vi "Digital In Test_TS_v2.vi"(8 "error in (no error)":errorcluster, 11 "ControlBoard VISA":refnum<visa-resource-name>="ControlBoard") -> (0 "error out":errorcluster, 2 "Message OUT":string, 3 "Result (bool)":bool)   [LabVIEW 2022 SP3]
uses:
  <vilib>/DAQmx/write.llb/DAQmx Write (Digital 1D Bool NChan 1Samp 1Line).vi
  <vilib>/DAQmx/miscellaneous.llb/DAQmx Fill In Error Info.vi
panel:
  in  "Message IN":string
  out "cDAQ DO Cmd":bool[](array[boolean])
  out "DI Reading":bool[](array[boolean])
  out "ControlBoard VISA Out":refnum<visa-resource-name>
  out "Result (color)":u32(colorbox)
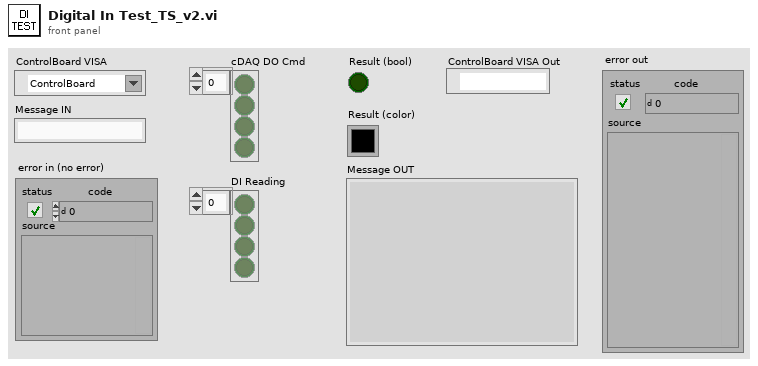
[diagram p1: front panel]
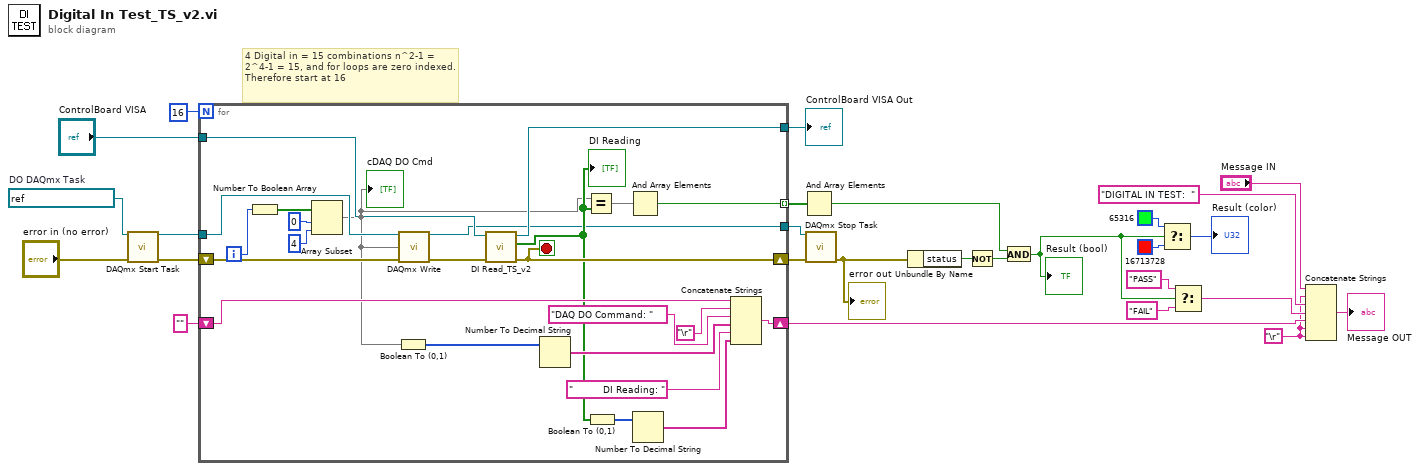
[diagram p0: block diagram]
diagram:
  w5 = refnum<k21> "BTS_DigitalOut"  # DO DAQmx Task
  w11 = "\r"
  # "4 Digital in = 15 combinations n^2-1 = 2^4-1 = 15, and for loops are zero indexed.  Therefore start at 16"
  n1 = call <vilib>:"DAQmx Start Task.vi"("task/channels in"=w5, "error in"="error in (no error)") -> ("task out"=w6:refnum<k21>, "error out"=w3:errorcluster)  [unwired: 12 in]
  n2 = for {
    N: 16 -> [_]
    shift-right: [w46] -> w2
    shift-left: w3 -> [w51]
    tunnel: [w50] -> w9
    tunnel: [w49] -> w21 mode=indexing
    shift-right: [w38] -> w16
    shift-left: "" -> [w37]
    tunnel: "ControlBoard VISA" -> [w31]
    tunnel: [w30] -> w7
    tunnel: w6 -> [w29]
    i -> [w47]
    stop <- w46 stop-if-true
    n3 = Number To Boolean Array(number=w47) -> (Boolean array=w33:bool[])
    n4 = Array Subset(array=w33, index=0, length=4) -> (w28:bool[])
    "cDAQ DO Cmd" <- w28
    n5 = Boolean To (0,1)(Boolean=w28) -> (0, 1=w40:i16[])
    n6 = call-poly <vilib>:"DAQmx Write.vi"("task/channels in"=w29, "data"=w28, "error in"=w51) -> ("task out"=w30:refnum<k21>, "error out"=w32:errorcluster)  [unwired: 10 in, 1 out]
    n7 = call "DI Read_TS_v2.vi"("error in (no error)"=w32, "ControlBoard VISA"=w31) -> ("error out"=w46:errorcluster, "DI Reading"=w36:bool[], "VISA Refnum out"=w50:refnum<visa-resource-name>)  [unwired: 6 in, 1 out]
    "DI Reading" <- w36
    n8 = Number To Decimal String(number=w40) -> (decimal integer string=w43:string[])  [unwired: 1 in]
    n9 = Equal?(x=w28, y=w36) -> (x = y?=w48:bool[])
    n10 = Boolean To (0,1)(Boolean=w36) -> (0, 1=w39:i16[])
    n11 = And Array Elements(Boolean array=w48) -> (logical AND=w49:bool)
    n12 = Number To Decimal String(number=w39) -> (decimal integer string=w45:string[])  [unwired: 1 in]
    n13 = Concatenate Strings(w37, "\r", "DAQ DO Command: ", w43, "          DI Reading: ", w45) -> (w38:string)
  }
  "ControlBoard VISA Out" <- w9
  n14 = And Array Elements(Boolean array=w21) -> (logical AND=w18:bool)
  n15 = call <vilib>:"DAQmx Stop Task.vi"("task/channels in"=w7, "error in"=w2) -> ("error out"=w1:errorcluster)  [unwired: 12 in, 1 out]
  "error out" <- w1
  n16 = Unbundle By Name(w1) -> ("status"=w20:bool)
  n17 = Not(x=w20) -> (.not. x?=w17:bool)
  n18 = And(x=w18, y=w17) -> (x .and. y?=w19:bool)
  "Result (bool)" <- w19
  n19 = Select(t=u32 65316 ("Result (color)"), s=w19, f=u32 16713728 ("Result (color)")) -> (s? t:f=→"Result (color)":u32)
  n20 = Select(t="PASS", s=w19, f="FAIL") -> (s? t:f=w13:string)
  n21 = Concatenate Strings("Message IN", w11, "DIGITAL IN TEST:  ", w13, w16, w11, w11) -> (→"Message OUT":string)
